vi "Quantronix-command-file-parser.vi"(8 "Move speed [mm/s]":i32=500, 9 "Scan speed [mm/s]":i32=141, 11 "Scan pattern file path":path=path "C:/Users/Christoph/Work/D.3 Scanning patterns/Command files/2013-08 Scan pattern comparison/patterns_304Sub_14x4_Mar8-1a - Copy.co") -> (0 "Ycoors":dbl[](array[numeric]), 1 "Xcoors":dbl[](array[numeric]), 2 "Time":dbl[](array[numeric]), 3 "error out":errorcluster, 4 "LaserONout":bool[](array[boolean]), 5 "Speeds":dbl[](array[numeric]), 7 "Lines":i32[](array[numeric]))   [LabVIEW 2013, in "CameraVision.lvlib" / "CV-Mapping.lvclass"]
uses:
  CV-Mapping.lvclass
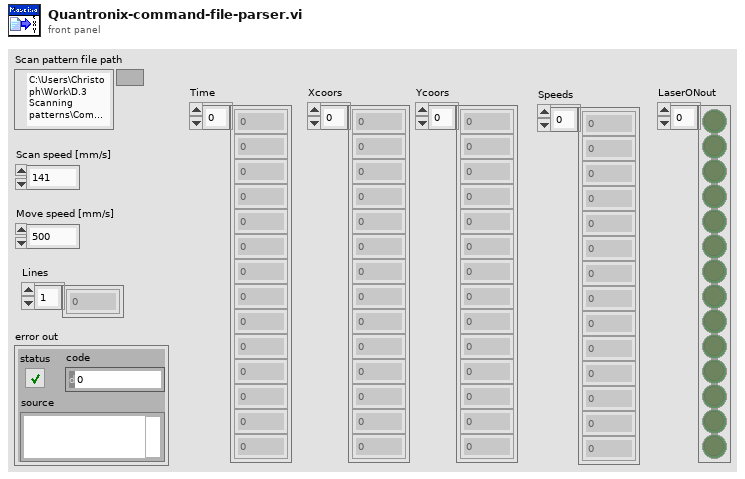
[diagram p1: front panel]
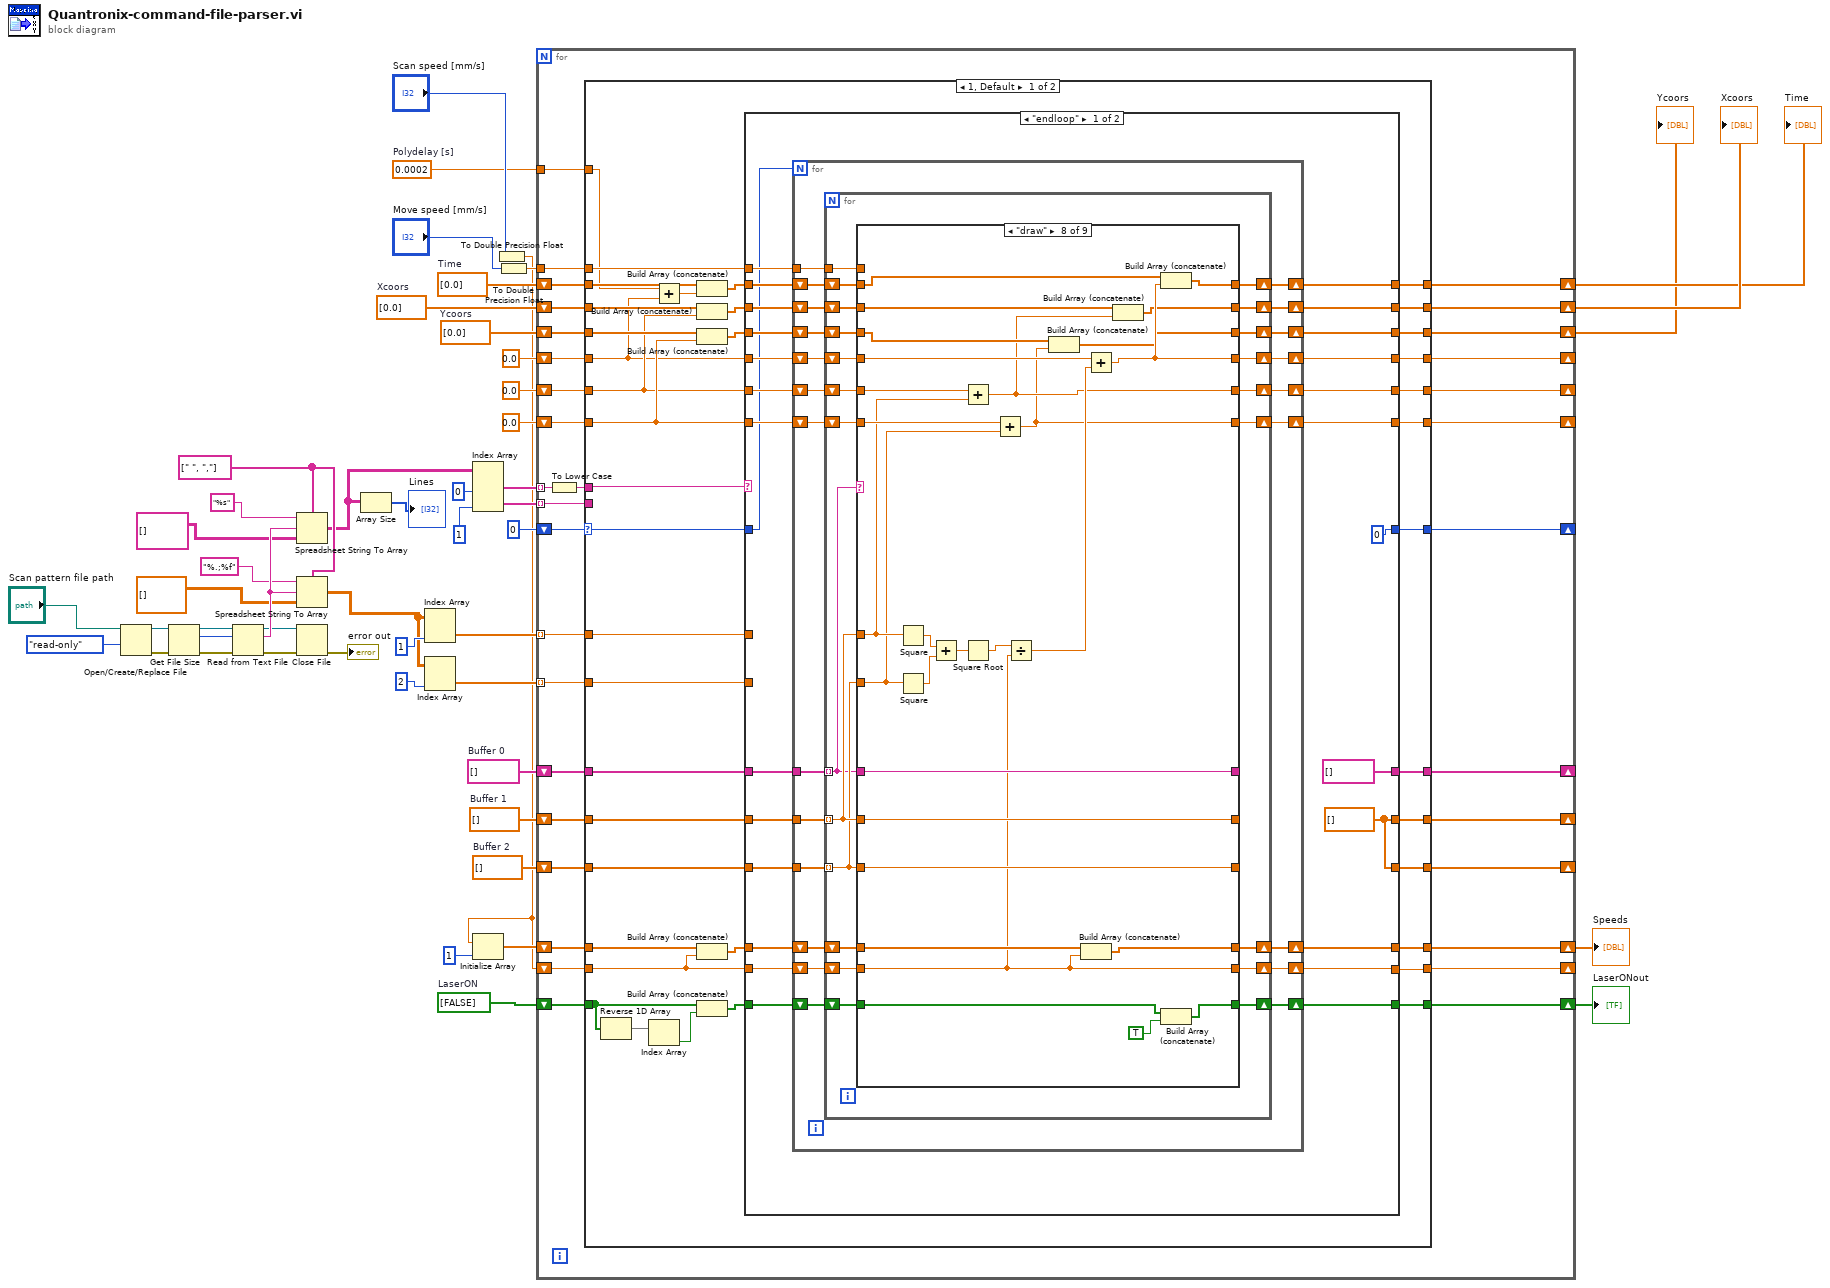
[diagram p0: block diagram]
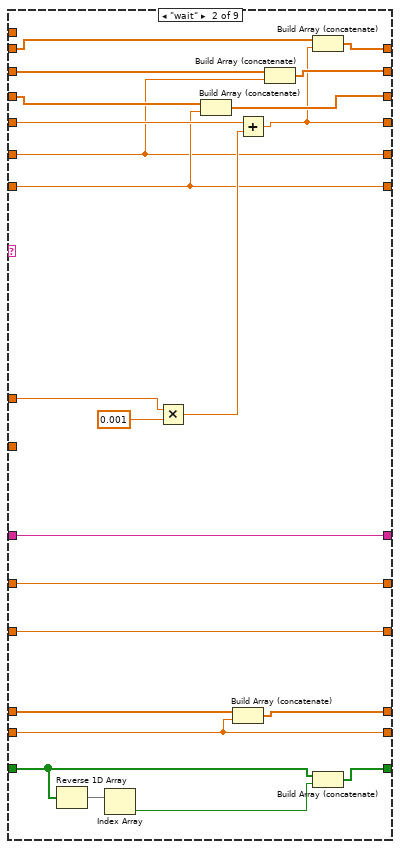
[diagram p3: hidden frame]
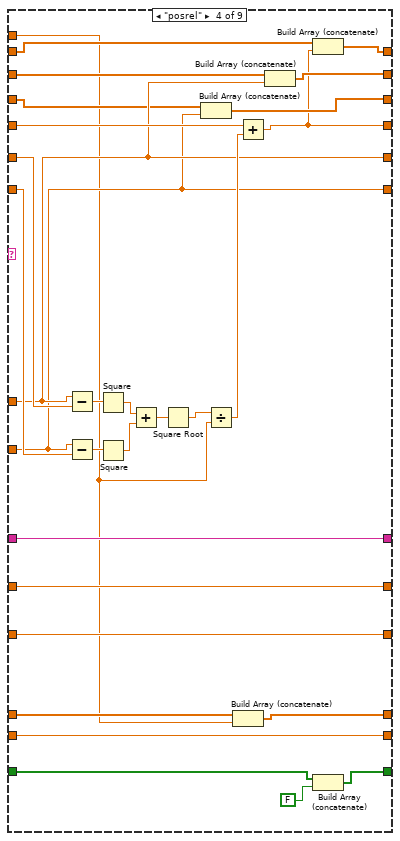
[diagram p5: hidden frame]
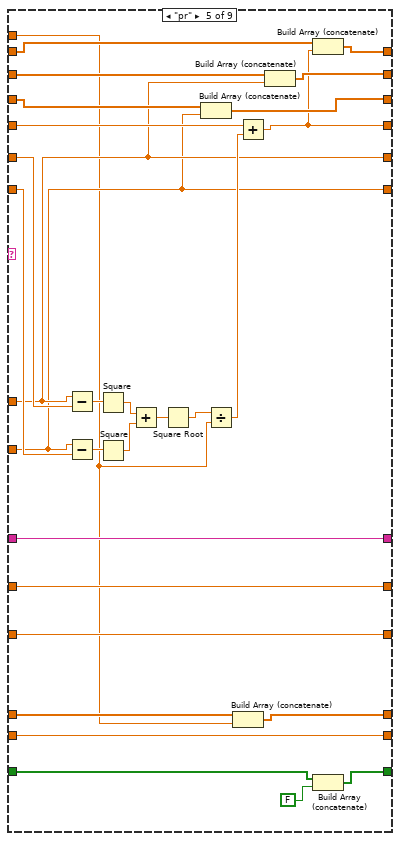
[diagram p6: hidden frame]
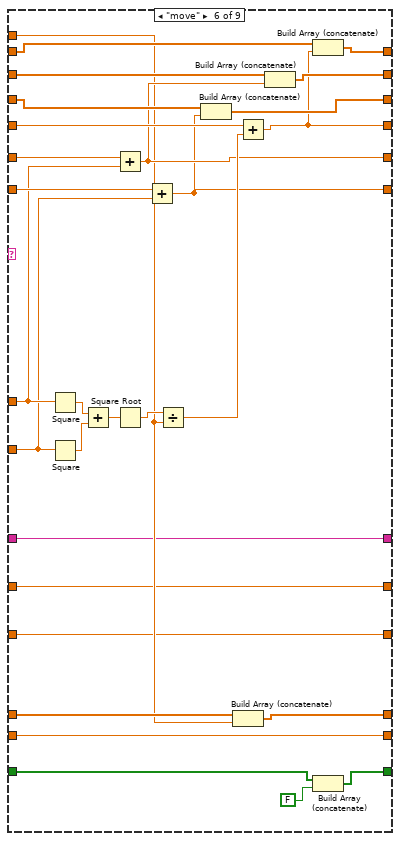
[diagram p7: hidden frame]
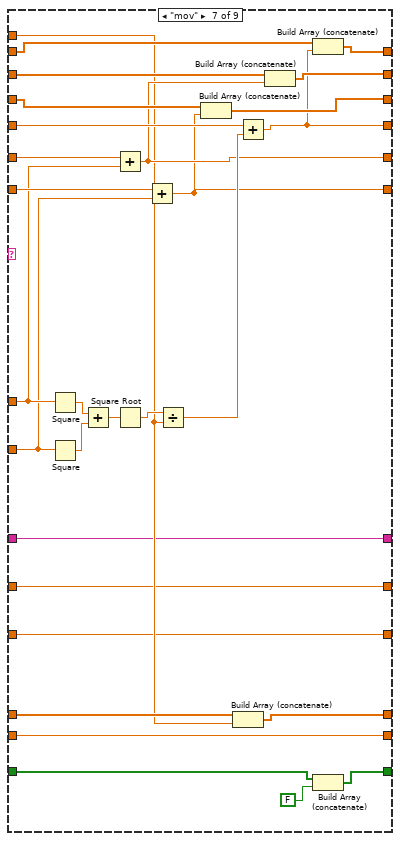
[diagram p8: hidden frame]
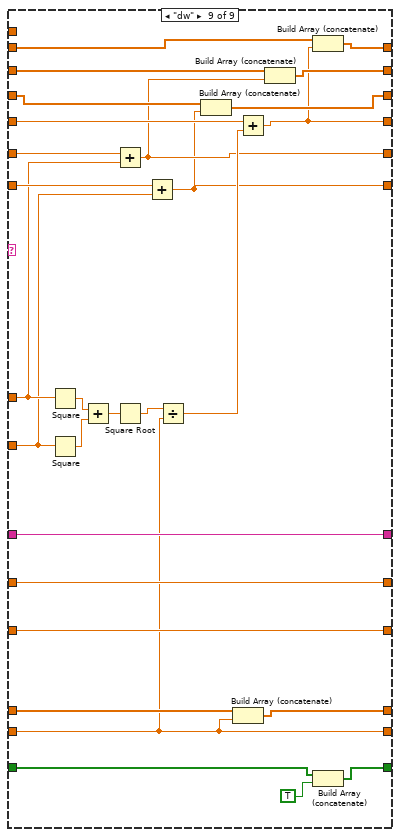
[diagram p9: hidden frame]
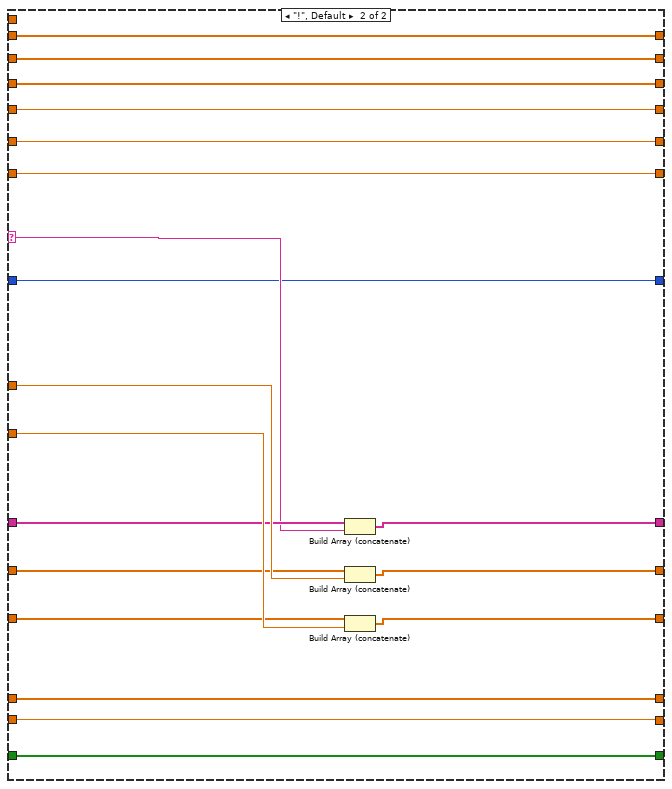
[diagram p10: hidden frame]
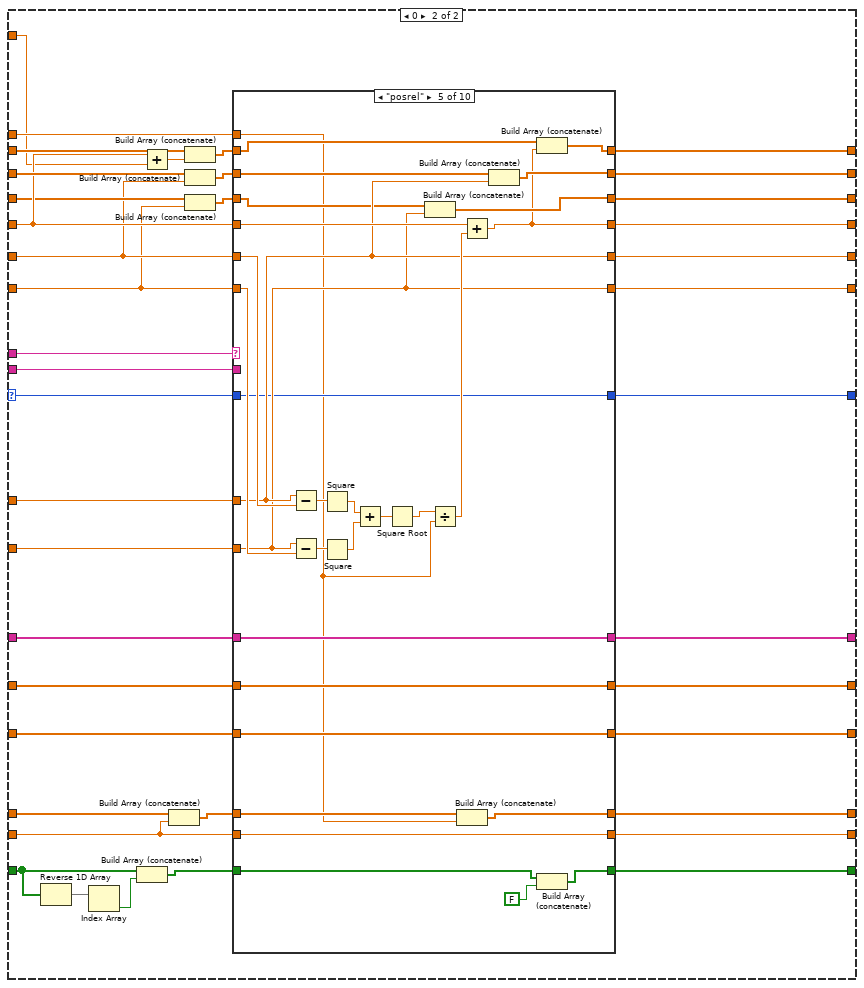
[diagram p11: hidden frame]
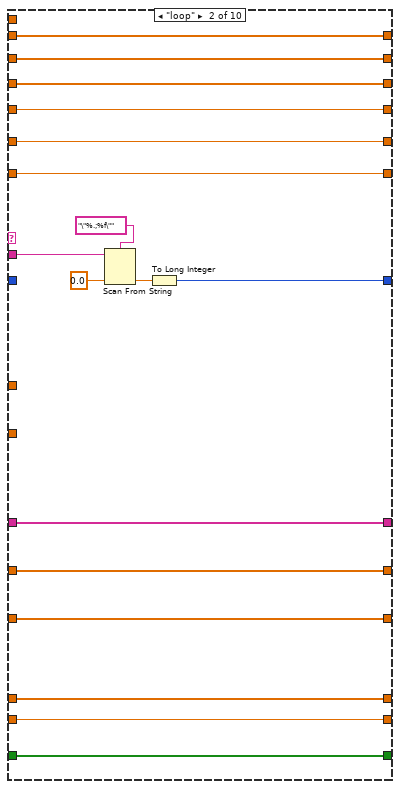
[diagram p13: hidden frame]
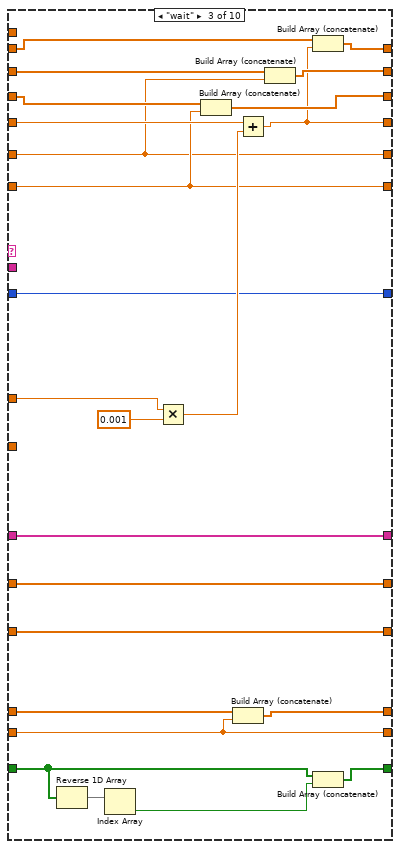
[diagram p14: hidden frame]
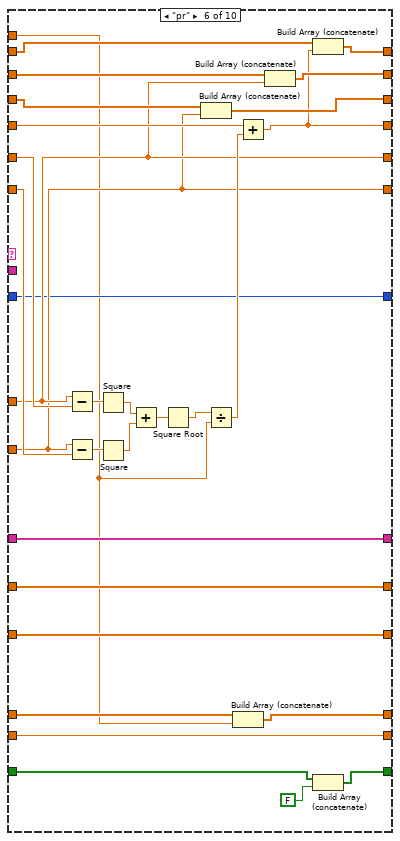
[diagram p16: hidden frame]
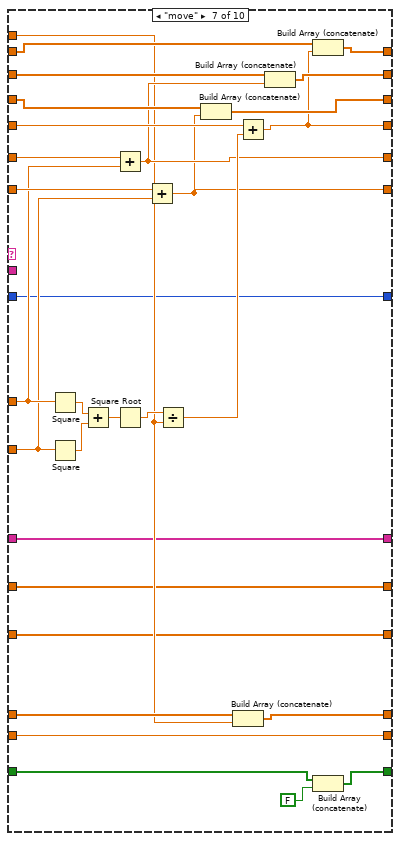
[diagram p17: hidden frame]
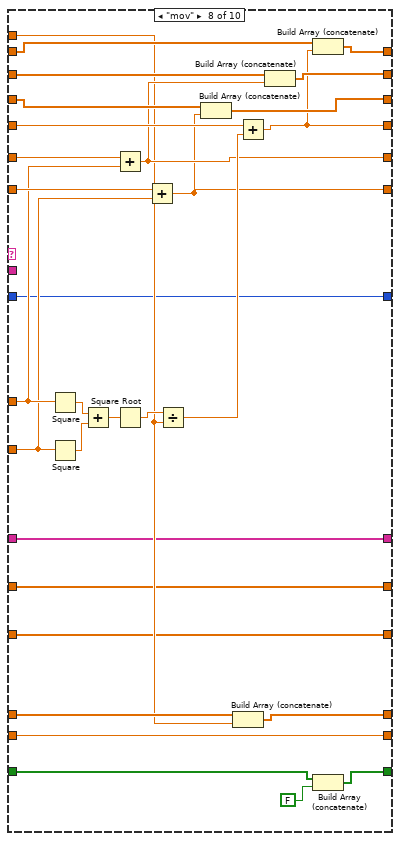
[diagram p18: hidden frame]
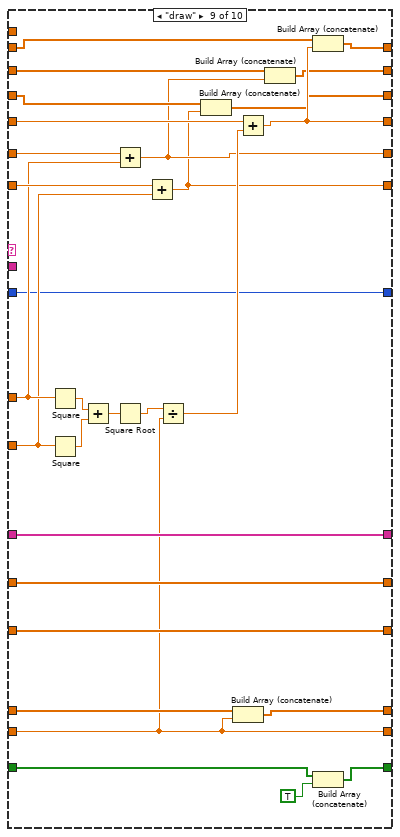
[diagram p19: hidden frame]
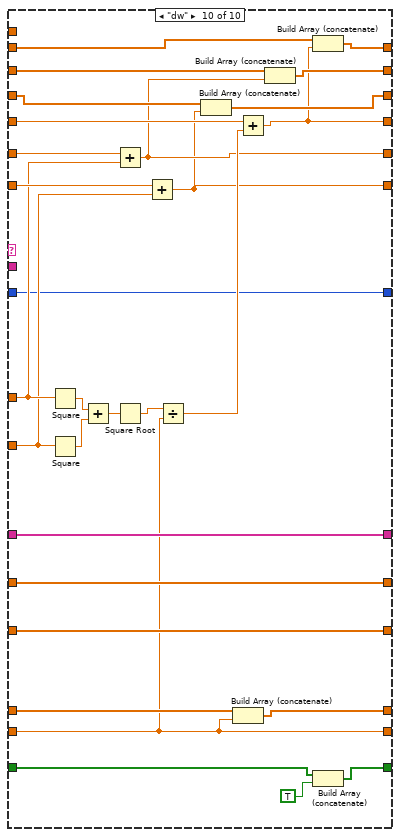
[diagram p20: hidden frame]
diagram:
  w1 = 0.0002  # Polydelay [s]
  w9 = string[] []  # Buffer 0
  w7 = dbl[] []  # Buffer 2
  w8 = dbl[] []  # Buffer 1
  w15 = bool[] [FALSE]  # LaserON
  w46 = dbl[] [0.0]  # Ycoors
  w45 = dbl[] [0.0]  # Xcoors
  w44 = dbl[] [0.0]  # Time
  w32 = string[] [" ", ","]
  n1 = Open/Create/Replace File(file path (use dialog)="Scan pattern file path", access (0:read/write)=enum16{"read/write", "read-only", "write-only"}."read-only") -> (refnum out=w21:refnum<file>, error out=w24:errorcluster)  [unwired: 4 in, 1 out]
  n2 = Get File Size(file=w21, error in=w24) -> (refnum out=w18:refnum<file>, size (in bytes)=w19:i64, 0:w20:errorcluster)
  n3 = Read from Text File(file (use dialog)=w18, count=w19, error in=w20) -> (refnum out=w22:refnum<file>, text=w28:string, error out=w23:errorcluster)  [unwired: 2 out]
  n4 = Spreadsheet String To Array(delimiter (Tab)=w32, format string="%s" ("delimiter (Tab)"), spreadsheet string=w28, array type (2D Dbl)=string[][] []) -> (array=w13:string[][])
  n5 = Spreadsheet String To Array(delimiter (Tab)=w32, format string="%.;%f", spreadsheet string=w28, array type (2D Dbl)=dbl[][] []) -> (array=w34:dbl[][])
  n6 = Close File(refnum=w22, error in=w23) -> (error out=→"error out":errorcluster)  [unwired: 1 out]
  n7 = Array Size(array=w13) -> (size(s)=→"Lines":i32[])
  n8 = Index Array(array=w34, index (col)=1 ("index")) -> (element=w33:dbl[])  [unwired: 1 in]
  n9 = Index Array(array=w34, index (col)=2 ("length")) -> (element=w35:dbl[])  [unwired: 1 in]
  n10 = Index Array(array=w13, index (col) #1=0 ("disabled index (col)"), index (col) #2=1 ("index (col)")) -> (element #1=w39:string[], element #2=w10:string[])  [unwired: 2 in]
  n11 = To Double Precision Float(number="Scan speed [mm/s]") -> (double precision float=w2:dbl)
  n12 = Initialize Array(w2, 1 ("dimension size")) -> (w4:dbl[])
  n13 = To Double Precision Float(number="Move speed [mm/s]") -> (double precision float=w12:dbl)
  n14 = for {
    tunnel: w33 -> [w76] mode=indexing
    tunnel: w35 -> [w75] mode=indexing
    tunnel: w39 -> [w83] mode=indexing
    shift-right: [w79] -> _
    shift-left: 0.0 -> [w80]
    shift-right: [w78] -> _
    shift-left: 0.0 -> [w81]
    shift-right: [w77] -> _
    shift-left: 0.0 -> [w82]
    shift-right: [w69] -> w48
    shift-left: w46 -> [w72]
    shift-right: [w70] -> w50
    shift-left: w45 -> [w73]
    shift-right: [w71] -> w49
    shift-left: w44 -> [w74]
    tunnel: w12 -> [w68]
    shift-right: [w66] -> w14
    shift-left: w15 -> [w67]
    shift-right: [w64] -> w5
    shift-left: w4 -> [w65]
    shift-right: [w62] -> _
    shift-left: w2 -> [w63]
    tunnel: w10 -> [w61] mode=indexing
    shift-right: [w54] -> _
    shift-left: w9 -> [w59]
    shift-right: [w53] -> _
    shift-left: w8 -> [w58]
    shift-right: [w52] -> _
    shift-left: w7 -> [w57]
    shift-right: [w56] -> _
    shift-left: 0 ("default value 1") -> [w55]
    tunnel: w1 -> [w51]
    n15 = To Lower Case(string=w83) -> (all lower case string=w60:string)
    n16 = case shown="1, Default" w55 {
      selector: w55 -> [w113 w453]
      tunnel: w82 -> [w92 w443]
      tunnel: w81 -> [w94 w438]
      tunnel: w80 -> [w93 w439]
      tunnel: [w104 w470] -> w79
      tunnel: [w103 w469] -> w78
      tunnel: [w105 w468] -> w77
      tunnel: w76 -> [w121 w467]
      tunnel: w75 -> [w122 w466]
      tunnel: w74 -> [w100 w449]
      tunnel: w73 -> [w98 w445]
      tunnel: w72 -> [w97 w442]
      tunnel: [w108 w465] -> w71
      tunnel: [w107 w464] -> w70
      tunnel: [w106 w463] -> w69
      tunnel: w68 -> [w102 w447]
      tunnel: w67 -> [w86 w435]
      tunnel: [w111 w462] -> w66
      tunnel: w65 -> [w90 w433]
      tunnel: [w109 w461] -> w64
      tunnel: w63 -> [w88 w432]
      tunnel: [w110 w460] -> w62
      tunnel: w61 -> [_ w459]
      tunnel: w60 -> [w114 w458]
      tunnel: w59 -> [w120 w457]
      tunnel: w58 -> [w119 w456]
      tunnel: w57 -> [w118 w455]
      tunnel: [w112 w454] -> w56
      tunnel: [w115 w452] -> w54
      tunnel: [w116 w451] -> w53
      tunnel: [w117 w450] -> w52
      tunnel: w51 -> [w91 w440]
      frame 1, Default {
        n17 = Reverse 1D Array(array=w86) -> (reversed array=w87:bool[])
        n18 = Index Array(array=w87) -> (element=w85:bool)  [unwired: 1 in]
        n19 = Add(x=w91, y=w92) -> (x+y=w101:dbl)
        n20 = Build Array (concatenate)(w100, w101) -> (w99:dbl[])
        n21 = Build Array (concatenate)(w98, w93) -> (w95:dbl[])
        n22 = Build Array (concatenate)(w97, w94) -> (w96:dbl[])
        n23 = Build Array (concatenate)(w90, w88) -> (w89:dbl[])
        n24 = Build Array (concatenate)(w86, w85) -> (w84:bool[])
        n25 = case shown="\"endloop\"" w114 {
          selector: w114 -> [_ w422]
          tunnel: w122 -> [_ w430]
          tunnel: w121 -> [_ w429]
          tunnel: w120 -> [w139 w428]
          tunnel: w119 -> [w138 w427]
          tunnel: w118 -> [w137 w426]
          tunnel: [w132 w425] -> w117
          tunnel: [w132 w424] -> w116
          tunnel: [string[] [] w423] -> w115
          tunnel: w113 -> [w140 w421]
          tunnel: [0 w421] -> w112
          tunnel: [w129 w412] -> w111
          tunnel: w84 -> [w136 w412]
          tunnel: [w130 w413] -> w110
          tunnel: w88 -> [w135 w413]
          tunnel: [w131 w414] -> w109
          tunnel: w89 -> [w134 w414]
          tunnel: [w128 w420] -> w108
          tunnel: w99 -> [w147 w420]
          tunnel: [w127 w419] -> w107
          tunnel: w95 -> [w146 w419]
          tunnel: [w126 w418] -> w106
          tunnel: w96 -> [w145 w418]
          tunnel: [w125 w417] -> w105
          tunnel: w92 -> [w144 w417]
          tunnel: [w124 w416] -> w104
          tunnel: w93 -> [w143 w416]
          tunnel: [w123 w415] -> w103
          tunnel: w94 -> [w142 w415]
          tunnel: w102 -> [w141 _]
          frame "endloop" {
            w132 = dbl[] []
            n26 = for {
              N: w140 -> [_]
              shift-right: [w154] -> w128
              shift-left: w147 -> [w170]
              shift-right: [w153] -> w127
              shift-left: w146 -> [w169]
              shift-right: [w152] -> w126
              shift-left: w145 -> [w168]
              shift-right: [w151] -> w125
              shift-left: w144 -> [w167]
              shift-right: [w150] -> w124
              shift-left: w143 -> [w166]
              shift-right: [w149] -> w123
              shift-left: w142 -> [w165]
              tunnel: w141 -> [w164]
              tunnel: w139 -> [w163]
              tunnel: w138 -> [w162]
              tunnel: w137 -> [w161]
              shift-right: [w157] -> w131
              shift-left: w134 -> [w158]
              shift-right: [w156] -> w130
              shift-left: w135 -> [w159]
              shift-right: [w155] -> w129
              shift-left: w136 -> [w160]
              n27 = for {
                shift-right: [w176] -> w154
                shift-left: w170 -> [w192]
                shift-right: [w175] -> w153
                shift-left: w169 -> [w191]
                shift-right: [w174] -> w152
                shift-left: w168 -> [w190]
                shift-right: [w173] -> w151
                shift-left: w167 -> [w189]
                shift-right: [w172] -> w150
                shift-left: w166 -> [w188]
                shift-right: [w171] -> w149
                shift-left: w165 -> [w187]
                tunnel: w164 -> [w186]
                tunnel: w163 -> [w180] mode=indexing
                tunnel: w162 -> [w182] mode=indexing
                tunnel: w161 -> [w181] mode=indexing
                shift-right: [w179] -> w157
                shift-left: w158 -> [w183]
                shift-right: [w178] -> w156
                shift-left: w159 -> [w184]
                shift-right: [w177] -> w155
                shift-left: w160 -> [w185]
                n28 = case shown="\"draw\"" w180 {
                  tunnel: w189 -> [w202 w227 w237 w267 w296 w323 w352 w380 w408]
                  tunnel: w187 -> [w203 w217 w239 w259 w288 w325 w354 w382 w410]
                  tunnel: w188 -> [w204 w216 w238 w260 w289 w326 w355 w383 w411]
                  tunnel: [w204 w216 w238 w253 w281 w310 w339 w370 w395] -> w172
                  tunnel: [w203 w217 w239 w252 w280 w309 w338 w369 w394] -> w171
                  tunnel: [w202 w219 w237 w250 w279 w308 w337 w368 w393] -> w173
                  tunnel: w182 -> [_ w214 w233 w253 w281 w321 w350 w378 w406]
                  tunnel: w181 -> [_ _ _ w252 w280 w320 w349 w377 w405]
                  tunnel: w192 -> [w201 w222 w231 w255 w284 w311 w342 w373 w398]
                  tunnel: w191 -> [w200 w221 w230 w254 w283 w312 w341 w372 w397]
                  tunnel: w190 -> [w199 w220 w229 w251 w282 w313 w340 w371 w396]
                  tunnel: [w201 w225 w231 w257 w287 w316 w345 w367 w401] -> w176
                  tunnel: [w200 w224 w230 w258 w286 w315 w344 w366 w400] -> w175
                  tunnel: [w199 w223 w229 w256 w285 w314 w343 w365 w399] -> w174
                  tunnel: w186 -> [_ _ _ w240 w269 w302 w330 _ _]
                  tunnel: w185 -> [w198 w212 w228 w248 w277 w306 w335 w363 w391]
                  tunnel: [w198 w218 w228 w249 w278 w307 w336 w364 w392] -> w177
                  tunnel: w183 -> [w196 w210 w232 w246 w275 w304 w333 w361 w389]
                  tunnel: [w196 w205 w232 w245 w274 w303 w332 w360 w388] -> w179
                  tunnel: [w197 w209 w233 w241 w270 w301 w331 w356 w384] -> w178
                  tunnel: w184 -> [w197 w209 _ w241 w270 w301 w331 w356 w384]
                  tunnel: w180 -> [w195 w208 w236 w244 w273 w300 w329 w359 w387]
                  tunnel: w182 -> [w194 w207 w235 w243 w272 w299 w328 w358 w386]
                  tunnel: w181 -> [w193 w206 w234 w242 w271 w298 w327 w357 w385]
                  tunnel: [w195 w208 w236 w244 w273 w300 w329 w359 w387] -> _
                  tunnel: [w194 w207 w235 w243 w272 w299 w328 w358 w386] -> _
                  tunnel: [w193 w206 w234 w242 w271 w298 w327 w357 w385] -> _
                  frame "!", Default {
                  }
                  frame "wait" {
                    n29 = Reverse 1D Array(array=w212) -> (reversed array=w213:bool[])
                    n30 = Index Array(array=w213) -> (element=w211:bool)  [unwired: 1 in]
                    n31 = Multiply(x=w214, y=0.001) -> (x*y=w226:dbl)
                    n32 = Build Array (concatenate)(w220, w217) -> (w223:dbl[])
                    n33 = Build Array (concatenate)(w210, w209) -> (w205:dbl[])
                    n34 = Add(x=w227, y=w226) -> (x+y=w219:dbl)
                    n35 = Build Array (concatenate)(w221, w216) -> (w224:dbl[])
                    n36 = Build Array (concatenate)(w222, w219) -> (w225:dbl[])
                    n37 = Build Array (concatenate)(w212, w211) -> (w218:bool[])
                  }
                  frame "speed" {
                  }
                  frame "posrel" {
                    n38 = Subtract(x=w253, y=w260) -> (x-y=w262:dbl)
                    n39 = Subtract(x=w252, y=w259) -> (x-y=w261:dbl)
                    n40 = Square(x=w262) -> (x^2=w265:dbl)
                    n41 = Square(x=w261) -> (x^2=w264:dbl)
                    n42 = Add(x=w265, y=w264) -> (x+y=w263:dbl)
                    n43 = Square Root(x=w263) -> (sqrt(x)=w268:dbl)
                    n44 = Build Array (concatenate)(w251, w252) -> (w256:dbl[])
                    n45 = Divide(x=w268, y=w240) -> (x/y=w266:dbl)
                    n46 = Build Array (concatenate)(w246, w240) -> (w245:dbl[])
                    n47 = Add(x=w267, y=w266) -> (x+y=w250:dbl)
                    n48 = Build Array (concatenate)(w254, w253) -> (w258:dbl[])
                    n49 = Build Array (concatenate)(w255, w250) -> (w257:dbl[])
                    n50 = Build Array (concatenate)(w248, FALSE) -> (w249:bool[])
                  }
                  frame "pr" {
                    n51 = Subtract(x=w281, y=w289) -> (x-y=w291:dbl)
                    n52 = Subtract(x=w280, y=w288) -> (x-y=w290:dbl)
                    n53 = Square(x=w291) -> (x^2=w294:dbl)
                    n54 = Square(x=w290) -> (x^2=w293:dbl)
                    n55 = Add(x=w294, y=w293) -> (x+y=w292:dbl)
                    n56 = Square Root(x=w292) -> (sqrt(x)=w297:dbl)
                    n57 = Build Array (concatenate)(w282, w280) -> (w285:dbl[])
                    n58 = Divide(x=w297, y=w269) -> (x/y=w295:dbl)
                    n59 = Build Array (concatenate)(w275, w269) -> (w274:dbl[])
                    n60 = Add(x=w296, y=w295) -> (x+y=w279:dbl)
                    n61 = Build Array (concatenate)(w283, w281) -> (w286:dbl[])
                    n62 = Build Array (concatenate)(w284, w279) -> (w287:dbl[])
                    n63 = Build Array (concatenate)(w277, FALSE) -> (w278:bool[])
                  }
                  frame "move" {
                    n64 = Square(x=w321) -> (x^2=w319:dbl)
                    n65 = Square(x=w320) -> (x^2=w318:dbl)
                    n66 = Add(x=w319, y=w318) -> (x+y=w317:dbl)
                    n67 = Add(x=w326, y=w321) -> (x+y=w310:dbl)
                    n68 = Square Root(x=w317) -> (sqrt(x)=w324:dbl)
                    n69 = Add(x=w325, y=w320) -> (x+y=w309:dbl)
                    n70 = Divide(x=w324, y=w302) -> (x/y=w322:dbl)
                    n71 = Build Array (concatenate)(w313, w309) -> (w314:dbl[])
                    n72 = Build Array (concatenate)(w304, w302) -> (w303:dbl[])
                    n73 = Add(x=w323, y=w322) -> (x+y=w308:dbl)
                    n74 = Build Array (concatenate)(w312, w310) -> (w315:dbl[])
                    n75 = Build Array (concatenate)(w311, w308) -> (w316:dbl[])
                    n76 = Build Array (concatenate)(w306, FALSE) -> (w307:bool[])
                  }
                  frame "mov" {
                    n77 = Square(x=w350) -> (x^2=w348:dbl)
                    n78 = Square(x=w349) -> (x^2=w347:dbl)
                    n79 = Add(x=w348, y=w347) -> (x+y=w346:dbl)
                    n80 = Add(x=w355, y=w350) -> (x+y=w339:dbl)
                    n81 = Square Root(x=w346) -> (sqrt(x)=w353:dbl)
                    n82 = Add(x=w354, y=w349) -> (x+y=w338:dbl)
                    n83 = Divide(x=w353, y=w330) -> (x/y=w351:dbl)
                    n84 = Build Array (concatenate)(w340, w338) -> (w343:dbl[])
                    n85 = Build Array (concatenate)(w333, w330) -> (w332:dbl[])
                    n86 = Add(x=w352, y=w351) -> (x+y=w337:dbl)
                    n87 = Build Array (concatenate)(w341, w339) -> (w344:dbl[])
                    n88 = Build Array (concatenate)(w342, w337) -> (w345:dbl[])
                    n89 = Build Array (concatenate)(w335, FALSE) -> (w336:bool[])
                  }
                  frame "draw" {
                    n90 = Square(x=w378) -> (x^2=w376:dbl)
                    n91 = Square(x=w377) -> (x^2=w375:dbl)
                    n92 = Add(x=w376, y=w375) -> (x+y=w374:dbl)
                    n93 = Add(x=w383, y=w378) -> (x+y=w370:dbl)
                    n94 = Square Root(x=w374) -> (sqrt(x)=w381:dbl)
                    n95 = Add(x=w382, y=w377) -> (x+y=w369:dbl)
                    n96 = Divide(x=w381, y=w356) -> (x/y=w379:dbl)
                    n97 = Build Array (concatenate)(w371, w369) -> (w365:dbl[])
                    n98 = Build Array (concatenate)(w361, w356) -> (w360:dbl[])
                    n99 = Add(x=w380, y=w379) -> (x+y=w368:dbl)
                    n100 = Build Array (concatenate)(w372, w370) -> (w366:dbl[])
                    n101 = Build Array (concatenate)(w373, w368) -> (w367:dbl[])
                    n102 = Build Array (concatenate)(w363, TRUE) -> (w364:bool[])
                  }
                  frame "dw" {
                    n103 = Square(x=w406) -> (x^2=w404:dbl)
                    n104 = Square(x=w405) -> (x^2=w403:dbl)
                    n105 = Add(x=w404, y=w403) -> (x+y=w402:dbl)
                    n106 = Add(x=w411, y=w406) -> (x+y=w395:dbl)
                    n107 = Square Root(x=w402) -> (sqrt(x)=w409:dbl)
                    n108 = Add(x=w410, y=w405) -> (x+y=w394:dbl)
                    n109 = Divide(x=w409, y=w384) -> (x/y=w407:dbl)
                    n110 = Build Array (concatenate)(w396, w394) -> (w399:dbl[])
                    n111 = Build Array (concatenate)(w389, w384) -> (w388:dbl[])
                    n112 = Add(x=w408, y=w407) -> (x+y=w393:dbl)
                    n113 = Build Array (concatenate)(w397, w395) -> (w400:dbl[])
                    n114 = Build Array (concatenate)(w398, w393) -> (w401:dbl[])
                    n115 = Build Array (concatenate)(w391, TRUE) -> (w392:bool[])
                  }
                }
              }
            }
          }
          frame "!", Default {
            n116 = Build Array (concatenate)(w428, w422) -> (w423:string[])
            n117 = Build Array (concatenate)(w427, w429) -> (w424:dbl[])
            n118 = Build Array (concatenate)(w426, w430) -> (w425:dbl[])
          }
        }
      }
      frame 0 {
        n119 = Reverse 1D Array(array=w435) -> (reversed array=w437:bool[])
        n120 = Index Array(array=w437) -> (element=w436:bool)  [unwired: 1 in]
        n121 = Build Array (concatenate)(w435, w436) -> (w434:bool[])
        n122 = Add(x=w443, y=w440) -> (x+y=w448:dbl)
        n123 = Build Array (concatenate)(w433, w432) -> (w431:dbl[])
        n124 = Build Array (concatenate)(w449, w448) -> (w446:dbl[])
        n125 = Build Array (concatenate)(w445, w439) -> (w444:dbl[])
        n126 = Build Array (concatenate)(w442, w438) -> (w441:dbl[])
        n127 = case shown="\"posrel\"" w458 {
          tunnel: w443 -> [w481 w498 w524 w535 w566 w596 w624 w654 w683 w712]
          tunnel: w438 -> [w482 w499 w514 w537 w558 w588 w626 w656 w685 w714]
          tunnel: w439 -> [w483 w500 w513 w536 w559 w589 w627 w657 w686 w715]
          tunnel: [w483 w500 w513 w536 w552 w581 w611 w641 w673 w699] -> w470
          tunnel: [w482 w499 w514 w537 w551 w580 w610 w640 w672 w698] -> w469
          tunnel: [w481 w498 w516 w535 w549 w579 w609 w639 w671 w697] -> w468
          tunnel: w467 -> [_ _ w511 w527 w552 w581 w622 w652 w681 w710]
          tunnel: w466 -> [_ _ _ _ w551 w580 w621 w651 w680 w709]
          tunnel: w446 -> [w480 w497 w519 w530 w554 w584 w612 w644 w676 w702]
          tunnel: w444 -> [w479 w496 w518 w529 w553 w583 w613 w643 w675 w701]
          tunnel: w441 -> [w478 w495 w517 w528 w550 w582 w614 w642 w674 w700]
          tunnel: [w480 w497 w522 w530 w556 w587 w617 w647 w670 w705] -> w465
          tunnel: [w479 w496 w521 w529 w557 w586 w616 w646 w669 w704] -> w464
          tunnel: [w478 w495 w520 w528 w555 w585 w615 w645 w668 w703] -> w463
          tunnel: w447 -> [_ _ _ _ w538 w568 w603 w632 _ _]
          tunnel: w434 -> [w477 w494 w509 w525 w547 w577 w607 w637 w666 w695]
          tunnel: [w477 w494 w515 w525 w548 w578 w608 w638 w667 w696] -> w462
          tunnel: w431 -> [w475 w492 w507 w526 w545 w575 w605 w635 w664 w693]
          tunnel: [w475 w492 w506 w526 w544 w574 w604 w634 w663 w692] -> w461
          tunnel: [w476 w493 w505 w527 w539 w569 w602 w633 w658 w687] -> w460
          tunnel: w432 -> [w476 w493 w505 _ w539 w569 w602 w633 w658 w687]
          tunnel: w459 -> [_ w489 _ _ _ _ _ _ _ _]
          tunnel: w457 -> [w473 w486 w503 w533 w542 w572 w600 w630 w661 w690]
          tunnel: w456 -> [w472 w485 w502 w532 w541 w571 w599 w629 w660 w689]
          tunnel: w455 -> [w471 w484 w501 w531 w540 w570 w598 w628 w659 w688]
          tunnel: [w474 w487 w504 w534 w543 w573 w601 w631 w662 w691] -> w454
          tunnel: w453 -> [w474 _ w504 w534 w543 w573 w601 w631 w662 w691]
          tunnel: [w473 w486 w503 w533 w542 w572 w600 w630 w661 w690] -> w452
          tunnel: [w472 w485 w502 w532 w541 w571 w599 w629 w660 w689] -> w451
          tunnel: [w471 w484 w501 w531 w540 w570 w598 w628 w659 w688] -> w450
          frame "!", Default {
          }
          frame "loop" {
            n128 = Scan From String(format string="\"%.;%f\"", input string=w489, default 1=0.0 ("default value 1")) -> (output 1=w488:dbl)  [unwired: 2 in, 3 out]
            n129 = To Long Integer(number=w488) -> (32bit integer=w487:i32)
          }
          frame "wait" {
            n130 = Reverse 1D Array(array=w509) -> (reversed array=w510:bool[])
            n131 = Index Array(array=w510) -> (element=w508:bool)  [unwired: 1 in]
            n132 = Multiply(x=w511, y=0.001) -> (x*y=w523:dbl)
            n133 = Build Array (concatenate)(w517, w514) -> (w520:dbl[])
            n134 = Build Array (concatenate)(w507, w505) -> (w506:dbl[])
            n135 = Add(x=w524, y=w523) -> (x+y=w516:dbl)
            n136 = Build Array (concatenate)(w518, w513) -> (w521:dbl[])
            n137 = Build Array (concatenate)(w519, w516) -> (w522:dbl[])
            n138 = Build Array (concatenate)(w509, w508) -> (w515:bool[])
          }
          frame "speed" {
          }
          frame "posrel" {
            n139 = Subtract(x=w552, y=w559) -> (x-y=w561:dbl)
            n140 = Subtract(x=w551, y=w558) -> (x-y=w560:dbl)
            n141 = Square(x=w561) -> (x^2=w564:dbl)
            n142 = Square(x=w560) -> (x^2=w563:dbl)
            n143 = Add(x=w564, y=w563) -> (x+y=w562:dbl)
            n144 = Square Root(x=w562) -> (sqrt(x)=w567:dbl)
            n145 = Build Array (concatenate)(w550, w551) -> (w555:dbl[])
            n146 = Divide(x=w567, y=w538) -> (x/y=w565:dbl)
            n147 = Build Array (concatenate)(w545, w538) -> (w544:dbl[])
            n148 = Add(x=w566, y=w565) -> (x+y=w549:dbl)
            n149 = Build Array (concatenate)(w553, w552) -> (w557:dbl[])
            n150 = Build Array (concatenate)(w554, w549) -> (w556:dbl[])
            n151 = Build Array (concatenate)(w547, FALSE) -> (w548:bool[])
          }
          frame "pr" {
            n152 = Subtract(x=w581, y=w589) -> (x-y=w591:dbl)
            n153 = Subtract(x=w580, y=w588) -> (x-y=w590:dbl)
            n154 = Square(x=w591) -> (x^2=w594:dbl)
            n155 = Square(x=w590) -> (x^2=w593:dbl)
            n156 = Add(x=w594, y=w593) -> (x+y=w592:dbl)
            n157 = Square Root(x=w592) -> (sqrt(x)=w597:dbl)
            n158 = Build Array (concatenate)(w582, w580) -> (w585:dbl[])
            n159 = Divide(x=w597, y=w568) -> (x/y=w595:dbl)
            n160 = Build Array (concatenate)(w575, w568) -> (w574:dbl[])
            n161 = Add(x=w596, y=w595) -> (x+y=w579:dbl)
            n162 = Build Array (concatenate)(w583, w581) -> (w586:dbl[])
            n163 = Build Array (concatenate)(w584, w579) -> (w587:dbl[])
            n164 = Build Array (concatenate)(w577, FALSE) -> (w578:bool[])
          }
          frame "move" {
            n165 = Square(x=w622) -> (x^2=w620:dbl)
            n166 = Square(x=w621) -> (x^2=w619:dbl)
            n167 = Add(x=w620, y=w619) -> (x+y=w618:dbl)
            n168 = Add(x=w627, y=w622) -> (x+y=w611:dbl)
            n169 = Square Root(x=w618) -> (sqrt(x)=w625:dbl)
            n170 = Add(x=w626, y=w621) -> (x+y=w610:dbl)
            n171 = Divide(x=w625, y=w603) -> (x/y=w623:dbl)
            n172 = Build Array (concatenate)(w614, w610) -> (w615:dbl[])
            n173 = Build Array (concatenate)(w605, w603) -> (w604:dbl[])
            n174 = Add(x=w624, y=w623) -> (x+y=w609:dbl)
            n175 = Build Array (concatenate)(w613, w611) -> (w616:dbl[])
            n176 = Build Array (concatenate)(w612, w609) -> (w617:dbl[])
            n177 = Build Array (concatenate)(w607, FALSE) -> (w608:bool[])
          }
          frame "mov" {
            n178 = Square(x=w652) -> (x^2=w650:dbl)
            n179 = Square(x=w651) -> (x^2=w649:dbl)
            n180 = Add(x=w650, y=w649) -> (x+y=w648:dbl)
            n181 = Add(x=w657, y=w652) -> (x+y=w641:dbl)
            n182 = Square Root(x=w648) -> (sqrt(x)=w655:dbl)
            n183 = Add(x=w656, y=w651) -> (x+y=w640:dbl)
            n184 = Divide(x=w655, y=w632) -> (x/y=w653:dbl)
            n185 = Build Array (concatenate)(w642, w640) -> (w645:dbl[])
            n186 = Build Array (concatenate)(w635, w632) -> (w634:dbl[])
            n187 = Add(x=w654, y=w653) -> (x+y=w639:dbl)
            n188 = Build Array (concatenate)(w643, w641) -> (w646:dbl[])
            n189 = Build Array (concatenate)(w644, w639) -> (w647:dbl[])
            n190 = Build Array (concatenate)(w637, FALSE) -> (w638:bool[])
          }
          frame "draw" {
            n191 = Square(x=w681) -> (x^2=w679:dbl)
            n192 = Square(x=w680) -> (x^2=w678:dbl)
            n193 = Add(x=w679, y=w678) -> (x+y=w677:dbl)
            n194 = Add(x=w686, y=w681) -> (x+y=w673:dbl)
            n195 = Square Root(x=w677) -> (sqrt(x)=w684:dbl)
            n196 = Add(x=w685, y=w680) -> (x+y=w672:dbl)
            n197 = Divide(x=w684, y=w658) -> (x/y=w682:dbl)
            n198 = Build Array (concatenate)(w674, w672) -> (w668:dbl[])
            n199 = Build Array (concatenate)(w664, w658) -> (w663:dbl[])
            n200 = Add(x=w683, y=w682) -> (x+y=w671:dbl)
            n201 = Build Array (concatenate)(w675, w673) -> (w669:dbl[])
            n202 = Build Array (concatenate)(w676, w671) -> (w670:dbl[])
            n203 = Build Array (concatenate)(w666, TRUE) -> (w667:bool[])
          }
          frame "dw" {
            n204 = Square(x=w710) -> (x^2=w708:dbl)
            n205 = Square(x=w709) -> (x^2=w707:dbl)
            n206 = Add(x=w708, y=w707) -> (x+y=w706:dbl)
            n207 = Add(x=w715, y=w710) -> (x+y=w699:dbl)
            n208 = Square Root(x=w706) -> (sqrt(x)=w713:dbl)
            n209 = Add(x=w714, y=w709) -> (x+y=w698:dbl)
            n210 = Divide(x=w713, y=w687) -> (x/y=w711:dbl)
            n211 = Build Array (concatenate)(w700, w698) -> (w703:dbl[])
            n212 = Build Array (concatenate)(w693, w687) -> (w692:dbl[])
            n213 = Add(x=w712, y=w711) -> (x+y=w697:dbl)
            n214 = Build Array (concatenate)(w701, w699) -> (w704:dbl[])
            n215 = Build Array (concatenate)(w702, w697) -> (w705:dbl[])
            n216 = Build Array (concatenate)(w695, TRUE) -> (w696:bool[])
          }
        }
      }
    }
  }
  "Time" <- w49
  "Xcoors" <- w50
  "Ycoors" <- w48
  "LaserONout" <- w14
  "Speeds" <- w5
